vi "SubMotionMetric.vi"(8 "error in (no error)":errorcluster, 11 "AVI Path":path) -> (0 "error out":errorcluster, 1 "z displacement":sgl[](array[numeric]), 2 "y displacement":sgl[](array[numeric]), 3 "x displacement":sgl[](array[numeric]))   [LabVIEW 2014]
uses:
  <vilib>/vision/NI_Vision_Development_Module.lvlib
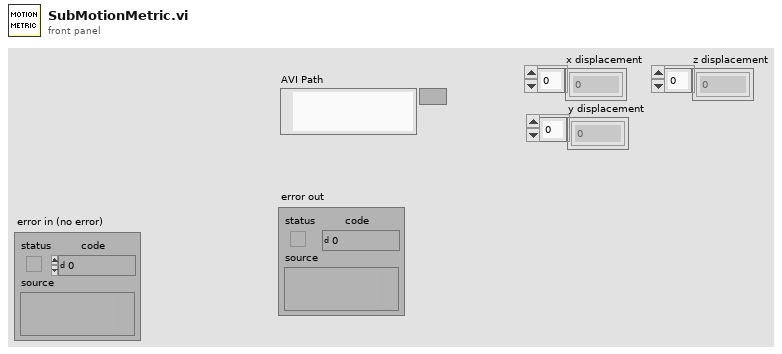
[diagram p1: front panel]
types:
  T1 = typedef "IMAQ Rectangle" = cluster{"Left":i32, "Top":i32, "Right":i32, "Bottom":i32, "Rotation":dbl}
  T2 = typedef "AviRefnum.ctl" = refnum<k1>
  T3 = typedef "ROI Descriptor" = cluster{"Global Rectangle":i32[], "Contours":cluster{"ID":enum32{"External", "Internal"}, "Type":u32, "Coordinates":i32[]}[]}
  T4 = typedef "IMAQ Image.ctl" = refnum<image>
  T5 = cluster{"Position":cluster{"x":sgl, "y":sgl}, "Angle":sgl, "Scale":sgl, "Score":sgl, "Bounding Box":cluster{"x":sgl, "y":sgl}[]}[]
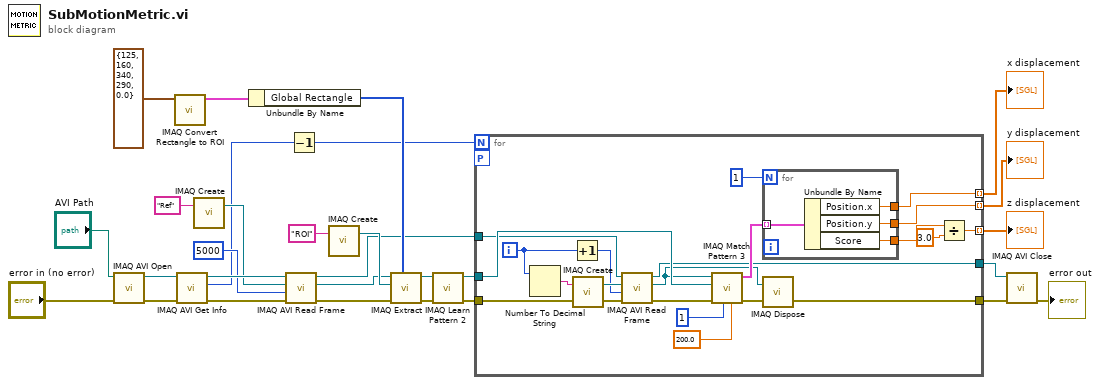
[diagram p0: block diagram]
diagram:
  n1 = call "IMAQ AVI Open"("error in (no error)"="error in (no error)", "AVI Path"="AVI Path") -> ("error out"=w19:errorcluster, "Avi Refnum"=w17:T2)  [unwired: 8 in]
  n2 = call "IMAQ Convert Rectangle to ROI"("Rectangle"=T1 {"Left"=125, "Top"=160, "Right"=340, "Bottom"=290, "Rotation"=0.0}) -> ("ROI Descriptor"=w21:T3)  [unwired: 8 in, 1 out]
  n3 = call "IMAQ AVI Get Info"("error in (no error)"=w19, "Avi Refnum"=w17) -> ("error out"=w18:errorcluster, "Number of Frames"=w10:u32, "Avi Refnum (duplicate)"=w16:T2)  [unwired: 5 in, 2 out]
  n4 = call "IMAQ Create"("Image Name"="Ref") -> ("New Image"=w15:T4)  [unwired: 4 in, 1 out]
  n5 = Unbundle By Name(w21) -> ("Global Rectangle"=w20:i32[])
  n6 = call "IMAQ AVI Read Frame"("error in (no error)"=w18, "Frame Number"=u32 5000, "Image"=w15, "Avi Refnum"=w16) -> ("error out"=w13:errorcluster, "Image Out"=w12:T4, "Avi Refnum (duplicate)"=w11:T2)  [unwired: 4 in, 1 out]
  n7 = Decrement(x=w10) -> (x-1=w9:u32)
  n8 = call "IMAQ Create"("Image Name"="ROI") -> ("New Image"=w28:T4)  [unwired: 4 in, 1 out]
  n9 = call "IMAQ Extract"("Optional Rectangle"=w20, "error in (no error)"=w13, "Image Dst"=w28, "Image Src"=w12) -> ("error out"=w26:errorcluster, "Image Dst Out"=w24:T4)  [unwired: 6 in]
  n10 = call "IMAQ Learn Pattern 2"("error in (no error)"=w26, "Image"=w24) -> ("error out"=w25:errorcluster, "Template Image Out"=w23:T4)  [unwired: 8 in]
  n11 = for {
    N: w9 -> [_]
    tunnel: w11 -> [w34]
    tunnel: w25 -> [w46]
    tunnel: w23 -> [w47]
    workers-P: _ -> [_]
    tunnel: [w40] -> w7
    tunnel: [w33] -> w6
    tunnel: [w32] -> w8 mode=indexing
    tunnel: [w31] -> w2 mode=indexing
    tunnel: [w30] -> w1 mode=indexing
    i -> [w42]
    n12 = Number To Decimal String(number=w42) -> (decimal integer string=w41:string)  [unwired: 1 in]
    n13 = Increment(x=w42) -> (x+1=w35:i32)
    n14 = call "IMAQ Create"("Image Name"=w41, "error in (no error)"=w46) -> ("New Image"=w36:T4, "error out"=w39:errorcluster)  [unwired: 3 in]
    n15 = call "IMAQ AVI Read Frame"("error in (no error)"=w39, "Frame Number"=w35, "Image"=w36, "Avi Refnum"=w34) -> ("error out"=w38:errorcluster, "Image Out"=w37:T4, "Avi Refnum (duplicate)"=w33:T2)  [unwired: 4 in, 1 out]
    n16 = call "IMAQ Match Pattern 3"("Minimum Match Score"=sgl 200.0, "Number of Matches Requested"=1, "error in (no error)"=w38, "Template Image"=w47, "Image"=w37) -> ("error out"=w43:errorcluster, "Matches"=w49:T5)  [unwired: 4 in, 1 out]
    n17 = for {
      N: 1 -> [_]
      tunnel: w49 -> [w55] mode=indexing
      tunnel: [w54] -> w32
      tunnel: [w53] -> w31
      tunnel: [w52] -> w44
      n18 = Unbundle By Name(w55) -> ("Position.x"=w54:sgl, "Position.y"=w53:sgl, "Score"=w52:sgl)
    }
    n19 = call "IMAQ Dispose"("Image"=w37, "error in (no error)"=w43) -> ("error out"=w40:errorcluster)  [unwired: 4 in]
    n20 = Divide(x=w44, y=sgl 3.0) -> (x/y=w30:sgl)
  }
  "x displacement" <- w8
  "y displacement" <- w2
  "z displacement" <- w1
  n21 = call "IMAQ AVI Close"("error in (no error)"=w7, "Avi Refnum"=w6) -> ("error out"=→"error out":errorcluster)  [unwired: 9 in]
